vi "Loop_ACT.vi"() -> ()   [LabVIEW 2017, in "Arm.lvlib"]
uses:
  Arm.lvlib
  _SHARE ALL/TypeDef Share All/CLUSTER_TalonInput.ctl
  _SHARE ALL/RoboRio Share All/SRX Share All/TypeDefs SRX/Cluster_SRX_PIDF.ctl
  _SHARE ALL/RoboRio Share All/SRX Share All/TypeDefs SRX/Cluster_SRX_Mode and Value.ctl
  System Drivers/Phoenix-LabVIEW/Motor Controller/Controls/CTRE_Phoenix_MotorControl_ControlMode.ctl
  _SHARE ALL/TypeDef Share All/CONTROL_PositonGraph.ctl
  CLUSTER_ACT_Lift Output.ctl
  _SHARE ALL/RoboRio Share All/SRX Share All/TypeDefs SRX/Cluster_SRX_Common Runtime Data.ctl
  _SHARE ALL/RoboRio Share All/SRX Share All/TypeDefs SRX/Cluster_SRX_Error Calculations.ctl
  _SHARE ALL/RoboRio Share All/SRX Share All/TypeDefs SRX/Cluster_SRX_Voltage Out Data.ctl
  _SHARE ALL/RoboRio Share All/SRX Share All/TypeDefs SRX/Cluster_SRX_Sensor Out Data.ctl
  _SHARE ALL/RoboRio Share All/SRX Share All/TypeDefs SRX/Cluster_SRX_F and R Limit Indicators.ctl
  Globals/Global_Device_IDs.vi
  _SHARE ALL/Global Share All/Global_STOP.vi
  Global_SM Write_Data Out.vi
  Global_ACT Write_Data Out.vi
panel:
  out "Rotation Output":T1 {"Common Runtime Data"."Temp" format="%.1f"; "Common Runtime Data"."Voltage"."Bus" format="%.3f"; "Common Runtime Data"."Voltage"."Output" format="%.3f"; "Common Runtime Data"."Voltage"."Percent" format="%.3f"; "Common Runtime Data"."Current" format="%.2f"}
  in  "Display Graph":bool
  out "Position Closed Loop Plots":T7
  out "Rotation Input":T8 {"SRXSet"."Mode" items=["PercentOutput"=0, "Position"=1, "Velocity"=2, "Current"=3, "Follower"=5, "MotionProfile"=6, "MotionMagic"=7, "MotionMagicArc"=8, "MotionProfileArc"=10, "Disabled"=15]}
  out "Cycle Time (S)":dbl format="%.3g"
  in  "Target Time(ms)":u32=50
  # "C"
  # "Units"
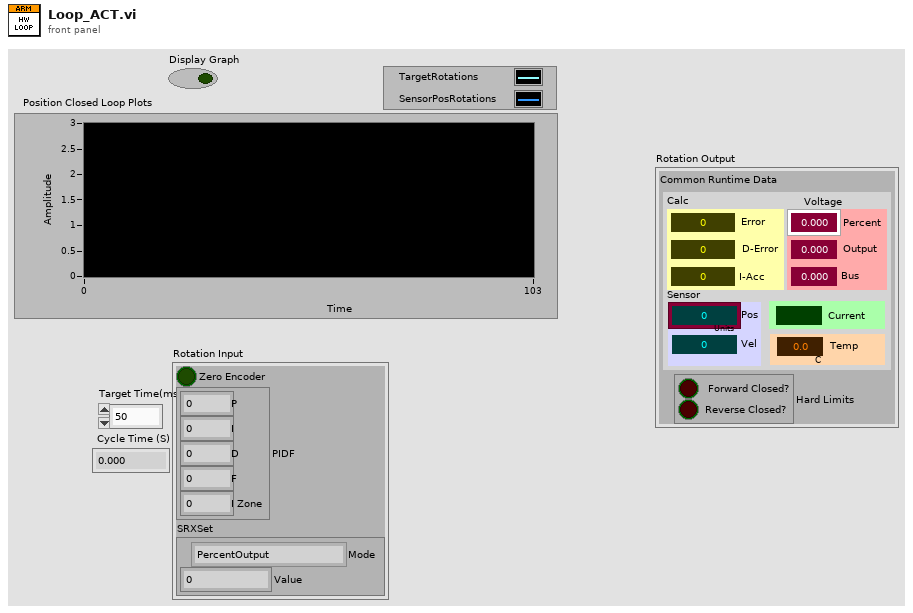
[diagram p1: front panel]
types:
  T1 = typedef "Arm.lvlib/CLUSTER_ACT_Lift Output.ctl" = cluster{"Common Runtime Data":T2, "Hard Limits":T6}
  T2 = typedef "Cluster_SRX_Common Runtime Data.ctl" = cluster{"Calc":T3, "Voltage ":T4, "Sensor":T5, "Current":dbl, "Temp":dbl}
  T3 = typedef "Cluster_SRX_Error Calculations.ctl" = cluster{"Error":i32, "D-Error":dbl, "I-Acc":dbl}
  T4 = typedef "Cluster_SRX_Voltage Out Data.ctl" = cluster{"Percent":dbl, "Output":dbl, "Bus":dbl}
  T5 = typedef "Cluster_SRX_Sensor Out Data.ctl" = cluster{"Pos":i32, "Vel":i32}
  T6 = typedef "Cluster_SRX_F and R Limit Indicators.ctl" = cluster{"Forward Closed?":bool, "Reverse Closed?":bool}
  T7 = typedef "CONTROL_PositonGraph.ctl" = cluster{dbl, "Position (Raw Sensor Units)":i32}
  T8 = typedef "CLUSTER_TalonInput.ctl" = cluster{"Zero Encoder":bool, "PIDF":T9, "SRXSet":T10}
  T9 = typedef "Cluster_SRX_PIDF.ctl" = cluster{"P":dbl, "I":dbl, "D":dbl, "F":dbl, "I Zone":dbl}
  T10 = typedef "Cluster_SRX_Mode and Value.ctl" = cluster{"Mode":T11, "Value":dbl}
  T11 = typedef "CTRE_Phoenix_MotorControl_ControlMode.ctl" = u16
  T12 = typedef "CLUSTER_Arm_Device_IDs.ctl" = cluster{"Master":T13, "Slave":T13, "Up PIDF":T9, "Down PIDF":T9}
  T13 = typedef "CLUSTER_Talon_Setup.ctl" = cluster{"Open Data":T14, "Current Config Data":T15, "Sensor Config":T16, "Hard Limits":T18, "Motion Magic Config Data":T20, "PIDF":T9, "Maximum Integral Accumulator Value":dbl, "AllowableClosedLoop":i32, "Limits":T21, "Output Config":T22}
  T14 = typedef "Cluster_SRX_OPEN Data.ctl" = cluster{"SRX ID":u8, "Invert Output":bool}
  T15 = typedef "Cluster_SRX_Current Config.ctl" = cluster{"Enable Current Limit?":bool, "Peak Current (Amps)":i32, "Peak Current Maximum Duration (ms)":i32, "Continuous Current Limit (Amps)":i32}
  T16 = typedef "Cluster_SRX_Sensor Config.ctl" = cluster{"Feedback Device":T17, "PhaseSensor":bool}
  T17 = typedef "CTRE_Phoenix_MotorControl_FeedbackDevice.ctl" = i8
  T18 = typedef "Cluster_SRX_Config Hard Limits.ctl" = cluster{"Fwd Enable":bool, "Rev Enable":bool, "Fwd NO-NC":T19, "Rev NO-NC":T19}
  T19 = typedef "CTRE_Phoenix_MotorControl_LimitSwitchNormal.ctl" = enum16{"Normally Open", "Normally Closed", "Disabled"}
  T20 = typedef "Cluster_SRX_Motion Magic Config Data.ctl" = cluster{"Cruise Velocity":i32, "Acceleration":i32}
  T21 = typedef "Cluster_SRX_Config Soft Limits.ctl" = cluster{"Max":i32, "Min":i32, "Max Enable":bool, "Min Enable":bool}
  T22 = typedef "Cluster_SRX_Config Voltage Output.ctl" = cluster{"Invert?":bool, "Neutral Mode":T23, "Deadband (-1to1)":dbl, "Ramp Time Off to Full (S)":dbl, "Peak  (-1to1)":T24, "Nominal  (-1to1)":T24}
  T23 = typedef "CTRE_Phoenix_MotorControl_NeutralMode.ctl" = enum8{"EEPROMSetting", "Override to Coast", "Override to Brake"}
  T24 = typedef "Cluster_SRX_Forward and Reverse.ctl" = cluster{"Forward":dbl, "Reverse":dbl}
  T25 = typedef "WPI_MotorControlDeviceRef.ctl" = cluster{"DeviceStatus":errorcluster, "Type":T26, "PWM":cluster{"PWM Channel":T27, "DeadBand":T28}, "CAN":cluster{"Device Number":u8, "SetOutput VI Ref":variant, "GetOutput VI Ref":variant, "Enable VI Ref":variant, "Disable VI Ref":variant, "Data":variant}, "Invert":bool, "DIO PWM":cluster{"PWM \"Enable\" Channel":T27, "DIOChannel":T29, "PWM Rate":dbl}}
  T26 = typedef "WPI_MotorControlType.ctl" = enum16{"PWM", "CAN", "DIO PWM"}
  T27 = typedef "FPGA_DIOPWMChannel.ctl" = enum8{"PWM 0", "PWM 1", "PWM 2", "PWM 3", "PWM 4", "PWM 5", "PWM 6", "PWM 7", "PWM 8", "PWM 9", "PWM MXP 0", "PWM MXP 1", "PWM MXP 2", "PWM MXP 3", "PWM MXP 4", "PWM MXP 5", "PWM MXP 6", "PWM MXP 7", "PWM MXP 8", "PWM MXP 9", "Invalid"}
  T28 = typedef "WPI_PWMDeadband.ctl" = cluster{"Name":string, "maxPositivePwm":i32, "minPositivePwm":i32, "centerPwm":i32, "maxNegativePwm":i32, "minNegativePwm":i32, "angularRange":u16}
  T29 = typedef "FPGA_DIOChannel.ctl" = enum8{"DIO 0", "DIO 1", "DIO 2", "DIO 3", "DIO 4", "DIO 5", "DIO 6", "DIO 7", "DIO 8", "DIO 9", "DIO MXP 0", "DIO MXP 1", "DIO MXP 2", "DIO MXP 3", "DIO MXP 4", "DIO MXP 5", "DIO MXP 6", "DIO MXP 7", "DIO MXP 8", "DIO MXP 9", "DIO MXP 10", "DIO MXP 11", "DIO MXP 12", "DIO MXP 13", "DIO MXP 14", "DIO MXP 15", "SPI Port CS1", "SPI Port CS2", "SPI Port CS3", "SPI Port MISO", "SPI Port MOSI", "Invalid"}
  T30 = cluster{"PhoenixMotorControlDevRef Out":T25, "Arm Output":T1, "Arm Input":T8, "Target Time(ms)":u32, "Current Time":timestamp, "Previous Time":timestamp, "Cycle Time (S)":dbl, "Last PID":T9}
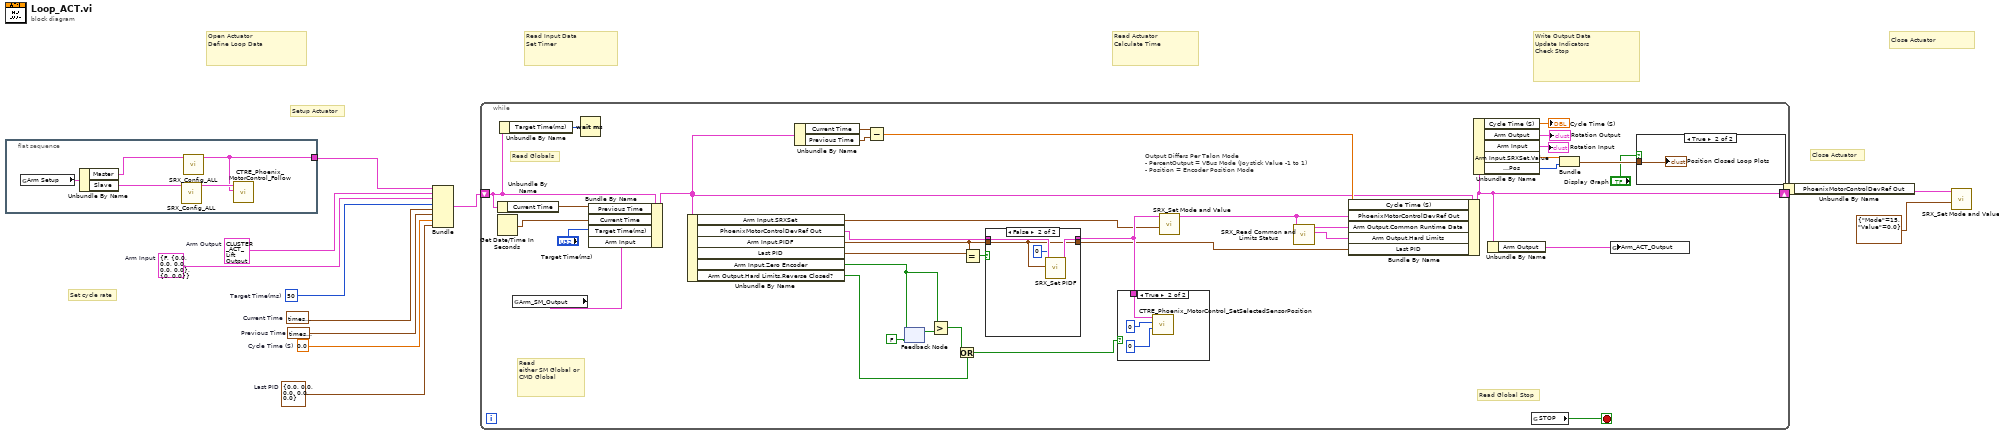
[diagram p0: block diagram]
diagram:
  w2 = T1 {"Common Runtime Data"={"Calc"={"Error"=0, "D-Error"=0.0, "I-Acc"=0.0}, "Voltage "={"Percent"=0.0, "Output"=0.0, "Bus"=0.0}, "Sensor"={"Pos"=0, "Vel"=0}, "Current"=0.0, "Temp"=0.0}, "Hard Limits"={"Forward Closed?"=FALSE, "Reverse Closed?"=FALSE}}  # Arm Output
  w4 = T9 {"P"=0.0, "I"=0.0, "D"=0.0, "F"=0.0, "I Zone"=0.0}  # Last PID
  w6 = T8 {"Zero Encoder"=FALSE, "PIDF"={"P"=0.0, "I"=0.0, "D"=0.0, "F"=0.0, "I Zone"=0.0}, "SRXSet"={"Mode"=0, "Value"=0.0}}  # Arm Input
  w7 = 0.0  # Cycle Time (S)
  w12 = timestamp(0 s since 1904-01-01)  # Previous Time
  w11 = timestamp(0 s since 1904-01-01)  # Current Time
  w10 = u32 50  # Target Time(ms)
  # "Close Actuator"
  # "Write Output Data\nUpdate Indicators\nCheck Stop"
  # "Read Actuator\nCalculate Time"
  # "Read Input Data\nSet Timer"
  # "Open Actuator\nDefine Loop Data"
  # "Set cycle rate"
  # "Close Actuator"
  # "Setup Actuator"
  n1 = flat-sequence {
    tunnel: [w13] -> w3
    frame #0 {
      n2 = global read "Global_Device_IDs.vi" "Arm Setup"() -> (w17:T12)
      n3 = Unbundle By Name(w17) -> ("Master"=w16:T13, "Slave"=w15:T13)
      n4 = call "SRX_Config_ALL.vi"("Talon Setup"=w15) -> ("PhoenixMotorControlDevRef Out"=w14:T25)  [unwired: 10 in]
      n5 = call "SRX_Config_ALL.vi"("Talon Setup"=w16) -> ("PhoenixMotorControlDevRef Out"=w13:T25)  [unwired: 10 in]
      n6 = call "CTRE_Phoenix_MotorControl_Follow.vi"("Master Controller To Follow"=w13, "PhoenixMotorControlDevRef"=w14) -> ()  [unwired: 8 in, 2 out]
    }
  }
  n7 = Bundle("PhoenixMotorControlDevRef Out"=w3, "Arm Output"=w2, "Arm Input"=w6, "Target Time(ms)"=w10, "Current Time"=w11, "Previous Time"=w12, "Cycle Time (S)"=w7, "Last PID"=w4) -> (w9:T30)  [unwired: 1 in]
  n8 = while {
    shift-right: [w45] -> w8
    shift-left: w9 -> [w47]
    stop <- w53 stop-if-true
    # "Output Differs Per Talon Mode\n- PercentOutput = VBus Mode (Joystick Value -1 to 1)\n- Position = Encoder Position Mode"
    # "Read\neither SM Global or CMD Global"
    # "Read Globals"
    # "Read Global Stop"
    n9 = Unbundle By Name(w47) -> ("Current Time"=w51:timestamp)
    n10 = Get Date/Time In Seconds() -> (seconds since 1Jan1904=w52:timestamp)
    n11 = Unbundle By Name(w47) -> ("Target Time(ms)"=w46:u32)
    n12 = global read "Global_SM Write_Data Out.vi" "Arm_SM_Output"() -> (w41:T8)
    n13 = Wait (ms)(milliseconds to wait=w46) -> ()  [unwired: 1 out]
    n14 = Bundle By Name(cluster=w47, "Previous Time"=w51, "Current Time"=w52, "Target Time(ms)"="Target Time(ms)", "Arm Input"=w41) -> (w36:T30)
    n15 = Unbundle By Name(w36) -> ("Arm Input.SRXSet"=w18:T10, "PhoenixMotorControlDevRef Out"=w35:T25, "Arm Input.PIDF"=w31:T9, "Last PID"=w32:T9, "Arm Input.Zero Encoder"=w27:bool, "Arm Output.Hard Limits.Reverse Closed?"=w19:bool)
    n16 = Unbundle By Name(w36) -> ("Current Time"=w50:timestamp, "Previous Time"=w49:timestamp)
    n17 = Subtract(x=w50, y=w49) -> (x-y=w43:dbl)
    n18 = feedback #1(FALSE) -> (w28:bool)
    n19 = feedback-in #1(w27) -> ()
    n20 = Greater?(x=w27, y=w28) -> (0:w21:bool)
    n21 = Or(x=w21, y=w19) -> (x .or. y?=w20:bool)
    n22 = Equal?(x=w31, y=w32) -> (x = y?=w30:bool)
    n23 = case shown="False" w30 {
      tunnel: w35 -> [w55 w59]
      tunnel: [w55 w58] -> w34
      tunnel: w31 -> [w54 w56]
      tunnel: [w54 w56] -> w23
      frame True {
      }
      frame False {
        n24 = call "SRX_Set PIDF.vi"("SlotIdx"=0 ("slotIdx"), "PIDF"=w56, "PhoenixMotorControlDevRef"=w59) -> ("PhoenixMotorControlDevRef Out"=w58:T25)  [unwired: 7 in, 1 out]
      }
    }
    n25 = case shown="True" w20 {
      tunnel: w34 -> [_ w63]
      frame False {
      }
      frame True {
        n26 = call "CTRE_Phoenix_MotorControl_SetSelectedSensorPosition.vi"("pidLoopIdx"=u32 0, "New Sensor Position"=0, "PhoenixMotorControlDevRef"=w63) -> ()  [unwired: 7 in, 2 out]
      }
    }
    n27 = call "SRX_Set Mode and Value.vi"("Mode And Value"=w18, "PhoenixMotorControlDevRef"=w34) -> ("PhoenixMotorControlDevRef Out"=w26:T25)  [unwired: 8 in, 1 out]
    n28 = call "SRX_Read Common and Limits Status.vi"("PhoenixMotorControlDevRef"=w26) -> ("Hard Limits Out"=w24:T6, "Common Runtime Data Out"=w25:T2)  [unwired: 8 in, 1 out]
    n29 = Bundle By Name(cluster=w36, "Cycle Time (S)"=w43, "PhoenixMotorControlDevRef Out"=w26, "Arm Output.Common Runtime Data"=w25, "Arm Output.Hard Limits"=w24, "Last PID"=w23) -> (w45:T30)
    n30 = Unbundle By Name(w45) -> ("Cycle Time (S)"=→"Cycle Time (S)":dbl, "Arm Output"=→"Rotation Output":T1, "Arm Input"=→"Rotation Input":T8, "Arm Input.SRXSet.Value"=w39:dbl, "Arm Output.Common Runtime Data.Sensor.Pos"=w38:i32)
    n31 = Unbundle By Name(w45) -> ("Arm Output"=w42:T1)
    n32 = global read "Global_STOP.vi" "STOP"() -> (w53:bool)
    n33 = Bundle("Value"=w39, "Pos"=w38) -> (w37:cluster{"Value":dbl, "Pos":i32})  [unwired: 1 in]
    n34 = global write "Global_ACT Write_Data Out.vi" "Arm_ACT_Output"(w42) -> ()
    n35 = case shown="True" "Display Graph" {
      tunnel: w37 -> [_ w60]
      frame False {
      }
      frame True {
        "Position Closed Loop Plots" <- w60
      }
    }
  }
  n36 = Unbundle By Name(w8) -> ("PhoenixMotorControlDevRef Out"=w5:T25)
  n37 = call "SRX_Set Mode and Value.vi"("Mode And Value"=T10 {"Mode"=15, "Value"=0.0}, "PhoenixMotorControlDevRef"=w5) -> ()  [unwired: 8 in, 2 out]
